vi "Get VI Data.vi"(8 "error in (no error)":errorcluster, 11 "VI in":refnum<vi>) -> (0 "error out":errorcluster, 1 "Conpane Image":T1, 2 "Array":string[](array[string]), 3 "VI out":refnum<vi>, 4 "Name":string, 5 "Panel":refnum<vi>)   [LabVIEW 2023, in "VI Properties Editor.lvlib"]
uses:
  VI Properties Editor.lvlib
  <vilib>/picture/picture.llb/imagedata.ctl
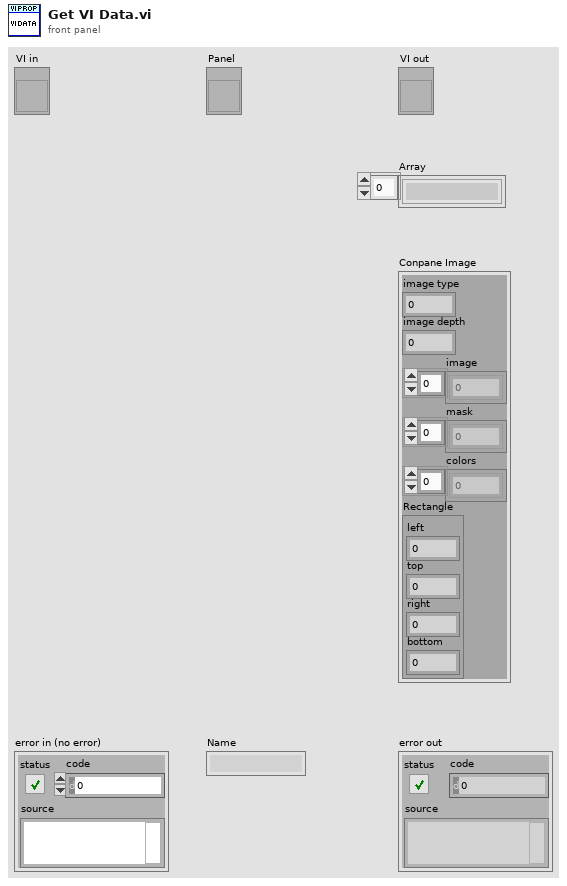
[diagram p1: front panel]
types:
  T1 = typedef "imagedata.ctl" = cluster{"image type":i32, "image depth":i32, "image":u8[], "mask":u8[], "colors":u32[], "Rectangle":cluster{"left":i16, "top":i16, "right":i16, "bottom":i16}}
  T2 = enum32{"invalid VI type", "Standard VI", "Control VI", "Global VI", "Polymorphic VI", "Configuration VI", "SubSystem", "Facade VI", "Method VI", "Statechart Diagram VI"}
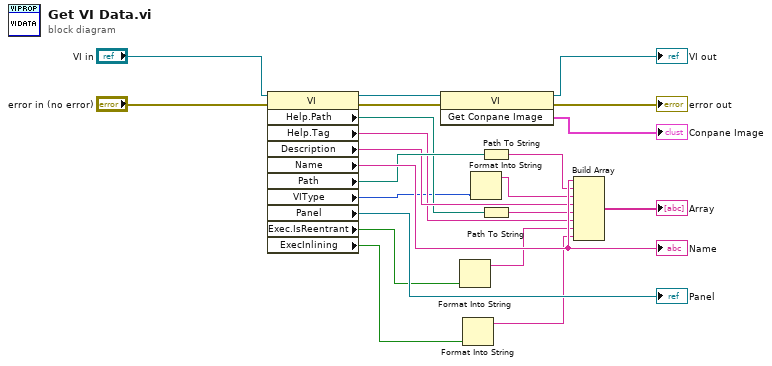
[diagram p0: block diagram]
diagram:
  n1 = property class="VI"(reference="VI in", error in="error in (no error)") -> (reference out=w10:refnum<vi>, error out=w11:errorcluster, "Help.Path"=w17:path, "Help.Tag"=w18:string, "Description"=w19:string, "Name"=w22:string, "Path"=w20:path, "VIType"=w8:T2, "Panel"=→"Panel":refnum<vi>, "Exec.IsReentrant"=w6:bool, "ExecInlining"=w4:bool)
  "Name" <- w22
  n2 = invoke class="VI" method="Get Conpane Image"(reference=w10, error in=w11) -> (reference out=→"VI out":refnum<vi>, error out=→"error out":errorcluster, "Get Conpane Image"=→"Conpane Image":T1)  [unwired: 1 in]
  n3 = Format Into String(w6) -> (resulting string=w5:string)  [unwired: 3 in, 1 out]
  n4 = Format Into String(w4) -> (resulting string=w3:string)  [unwired: 3 in, 1 out]
  n5 = Format Into String(w8) -> (resulting string=w7:string)  [unwired: 3 in, 1 out]
  n6 = Path To String(path=w20) -> (string=w16:string)
  n7 = Path To String(path=w17) -> (string=w15:string)
  n8 = Build Array(w22, w16, w7, w19, w15, w18, w5, w3) -> (→"Array":string[])
